vi "ToJson.vi"(8 "error in (no error)":errorcluster, 11 "Personnel in":refnum<class "Personnel.lvclass">) -> (0 "error out":errorcluster, 2 "PersonnelJson":string, 3 "Personnel out":refnum<class "Personnel.lvclass">)   [LabVIEW 2015, in "Personnel.lvclass"]
uses:
  Personnel.lvclass
  JsonCluster.ctl
  Personnel.lvclass/Personnel.ctl
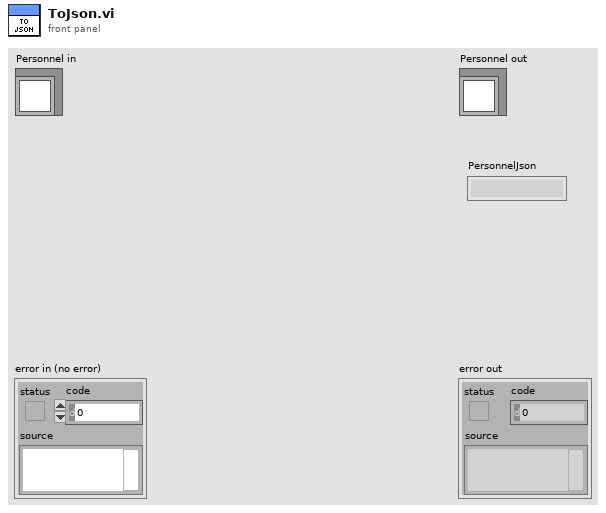
[diagram p1: front panel]
types:
  T1 = typedef "Personnel.lvclass/JsonCluster.ctl" = cluster{"Name":string, "Role":i32, "PUID":string, "Requests":string[]}
  T2 = typedef "Personnel.lvclass/PersonnelType.ctl" = enum16{"Nurse", "Doctor", "Cleanning", "Admin"}
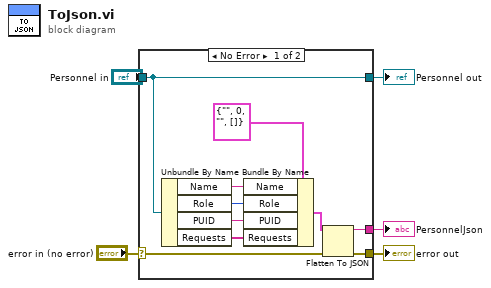
[diagram p0: block diagram]
diagram:
  n1 = case shown="No Error" "error in (no error)" {
    selector: "error in (no error)" -> [w7 w17]
    tunnel: [w6 w17] -> w4
    tunnel: [w9 w16] -> w2
    tunnel: "Personnel in" -> [w9 w16]
    tunnel: [w8 _] -> w1
    frame No Error {
      n2 = Unbundle By Name(w9) -> ("Name"=w14:string, "Role"=w13:T2, "PUID"=w12:string, "Requests"=w11:string[])
      n3 = Bundle By Name(cluster=T1 {"Name"="", "Role"=0, "PUID"="", "Requests"=[]} ("Personal Json"), "Name"=w14, "Role"=w13, "PUID"=w12, "Requests"=w11) -> (w10:T1)
      n4 = Flatten To JSON(anything=w10, error in (no error)=w7) -> (JSON string=w8:string, 11:w6:errorcluster)  [unwired: 1 in]
    }
    frame Error {
    }
  }
  "error out" <- w4
  "Personnel out" <- w2
  "PersonnelJson" <- w1
